vi "Last_L1_FileName_Result.vi"(7 "Function":T1(ring), 11 "FileName_in":string) -> (3 "FileName_Result?":bool)   [LabVIEW 2023]
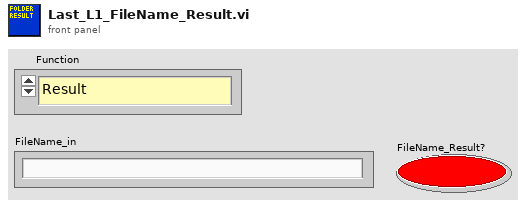
[diagram p1: front panel]
types:
  T1 = enum16{"Result", "Marker_1_26.5GHz", "Marker_2_28GHz", "Marker_3_29.5GHz", "Marker_4_31GHz"}
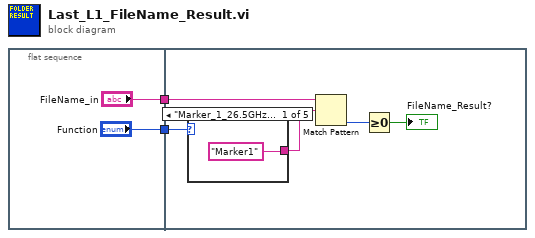
[diagram p0: block diagram]
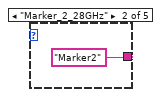
[diagram p2: hidden frame]
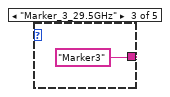
[diagram p3: hidden frame]
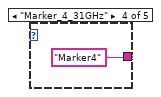
[diagram p4: hidden frame]
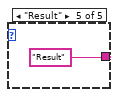
[diagram p5: hidden frame]
diagram:
  n1 = flat-sequence {
    tunnel: ["FileName_in"] -> w2
    tunnel: ["Function"] -> w1
    tunnel: w2 -> [w7]
    tunnel: w1 -> [w6]
    frame #0 {
    }
    frame #1 {
      n2 = case shown="\"Marker_1_26.5GHz\"" w6 {
        tunnel: ["Marker1" "Marker2" "Marker3" "Marker4" "Result"] -> w5
        frame "Marker_1_26.5GHz" {
        }
        frame "Marker_2_28GHz" {
        }
        frame "Marker_3_29.5GHz" {
        }
        frame "Marker_4_31GHz" {
        }
        frame "Result" {
        }
      }
      n3 = Match Pattern(string=w7, regular expression=w5) -> (offset past match=w8:i32)  [unwired: 1 in, 3 out]
      n4 = Greater Or Equal To 0?(x=w8) -> (x >= 0?=→"FileName_Result?":bool)
    }
  }
